vi "ReadMeasurementMetodo.vi"(6 "Measurement Type (0: Frequency)":i32(ring) items=["Frequency", "Mean", "Period", "Pulse Duty", "Peak to Peak", "Cycle RMS", "Minimum", "Maximum", "Rise Time", "Fall Time", "Positive Width", "Negative Width", "Amplitude", "Cycle Mean", "High", "Low", "Negative Duty", "Positive Overshoot", "Negative Overshoot", "Cursor Mean", "Burst Width", "Positive Pulse Count", "Negative Pulse Count", "Rising Edge Count", "Falling Edge Count", "Area", "Cycle Area", "RMS", "Cursor RMS"], 8 "error in (no error)":errorcluster, 9 "Channel (1: Channel 1)":i32(ring)=1 items=["Channel 1"=1, "Channel 2"=2, "Channel 3"=3, "Channel 4"=4], 11 "TektroniksTDS in":refnum<class "TektroniksTDS.lvclass">) -> (0 "error out":errorcluster, 1 "Units":string, 3 "TektroniksTDS out":refnum<class "TektroniksTDS.lvclass">, 4 "Measurement":dbl)   [LabVIEW 2020, in "TektroniksTDS.lvclass"]
uses:
  TektroniksTDS.lvclass
  TektroniksTDS.lvclass/TektroniksTDS.ctl
  <instrlib>/Tektronix TDS 200 1000 2000 Series/Tektronix TDS 200 1000 2000 Series.lvlib
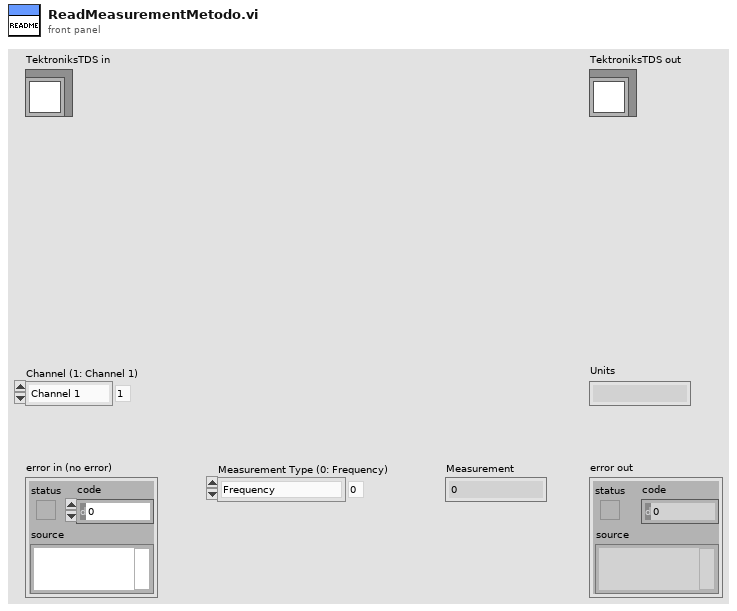
[diagram p1: front panel]
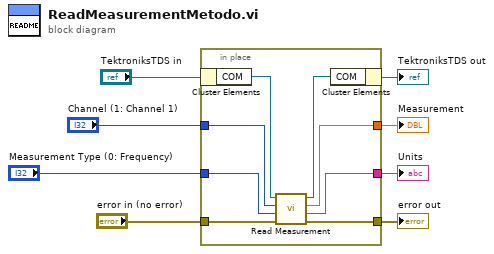
[diagram p0: block diagram]
diagram:
  n1 = in-place {
    in-place-border: "Channel (1: Channel 1)" -> [w14]
    in-place-border: "Measurement Type (0: Frequency)" -> [w13]
    in-place-border: [w12] -> w4
    in-place-border: [w11] -> w3
    in-place-border: [w10] -> w2
    in-place-border: "error in (no error)" -> [w9]
    n2 = in-place-cluster #1("TektroniksTDS in") -> ("COM"=w15:refnum<visa-resource-name>)
    n3 = call <instrlib>:"Read Measurement.vi"("error in (no error)"=w9, "Measurement Type (0: Frequency)"=w13, "Channel (1: Channel 1)"=w14, "VISA resource name"=w15) -> ("error out"=w12:errorcluster, "Units"=w10:string, "Measurement"=w11:dbl, "VISA resource name out"=w16:refnum<visa-resource-name>)  [unwired: 4 in]
    n4 = in-place-cluster #1("COM"=w16) -> (→"TektroniksTDS out":refnum<class "TektroniksTDS.lvclass">)
  }
  "error out" <- w4
  "Units" <- w2
  "Measurement" <- w3
